vi "Get_the_Process_Data.vi"(11 "Raw_Data":string[][](array[string])) -> (3 "Process_Data_Out":T1[][](array[typedef]))   [LabVIEW 2023]
doc: "Used to get the process data from the tsv file and build it as array of cluster."
uses:
  Control/Stage_Data.ctl
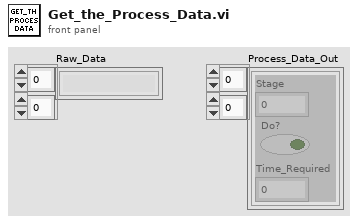
[diagram p1: front panel]
types:
  T1 = typedef "Stage_Data.ctl" = cluster{"Stage":i32, "Do?":bool, "Time_Required":i32}
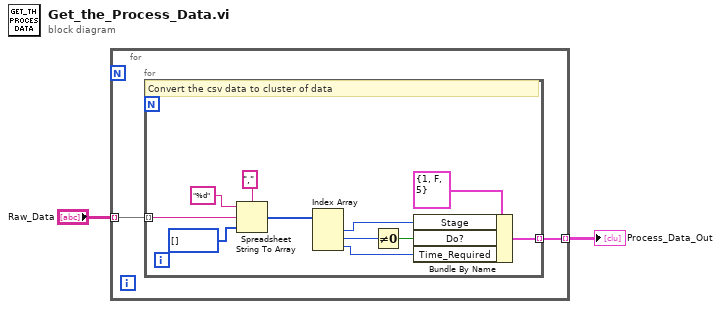
[diagram p0: block diagram]
diagram:
  n1 = for {
    tunnel: "Raw_Data" -> [w4] mode=indexing
    tunnel: [w3] -> w2 mode=indexing
    n2 = for {
      tunnel: w4 -> [w7] mode=indexing
      tunnel: [w8] -> w3 mode=indexing
      # "Convert the csv data to cluster of data"
      n3 = Spreadsheet String To Array(delimiter (Tab)=",", format string="%d", spreadsheet string=w7, array type (2D Dbl)=i32[] []) -> (array=w15:i32[])
      n4 = Index Array(array=w15) -> (element #1=w12:i32, element #2=w10:i32, element #3=w11:i32)  [unwired: 3 in]
      n5 = Not Equal To 0?(x=w10) -> (x != 0?=w9:bool)
      n6 = Bundle By Name(cluster=T1 {"Stage"=1, "Do?"=FALSE, "Time_Required"=5} ("Process_Details"), "Stage"=w12, "Do?"=w9, "Time_Required"=w11) -> (w8:T1)
    }
  }
  "Process_Data_Out" <- w2
